vi "dfd_Modify NStage MRate Modeling.vi"(8 "error in (no error)":errorcluster, 11 "multirate filters in":T1[](array[typedef]) {"mMRate_SumWl" min=1 max=32 step=1; "mMRate_InputIwl" min=1 max=32 step=1; "mMRate_GainWl" min=1 max=32 step=1; "mMRate_OutputWl" min=1 max=32 step=1; "mMRate_InputWl" min=1 max=32 step=1; "mMRate_CoefWl" min=1 max=32 step=1; "mMRate_Mode" items=["Default"=-1, "No Rate Change"=0, "Interpolation"=1, "Decimation"=2, "Interpolated"=3, "Rational"=4]}) -> (0 "error out":errorcluster, 3 "multirate filters out":T1[](array[typedef]) {"mMRate_SumWl" min=1 max=32 step=1; "mMRate_InputIwl" min=1 max=32 step=1; "mMRate_GainWl" min=1 max=32 step=1; "mMRate_OutputWl" min=1 max=32 step=1; "mMRate_InputWl" min=1 max=32 step=1; "mMRate_CoefWl" min=1 max=32 step=1; "mMRate_Mode" items=["Default"=-1, "No Rate Change"=0, "Interpolation"=1, "Decimation"=2, "Interpolated"=3, "Rational"=4]})   [LabVIEW 2017, in "NI_DigFilter_FXP.lvlib"]
uses:
  <vilib>/addons/Digital Filter Design/NI_DigFilter_FXP.lvlib
  <vilib>/addons/Digital Filter Design/_Objects.llb/DFD Multirate Filter Obj.ctl
  <vilib>/addons/Digital Filter Design/_Objects.llb/DFD Multirate Mode.ctl
  <vilib>/addons/Digital Filter Design/_Objects.llb/DFD Coef Norm Type.ctl
  <vilib>/addons/Digital Filter Design/_Objects.llb/DFD Round-off Mode.ctl
  <vilib>/addons/Digital Filter Design/_Objects.llb/DFD FXP MRate Multiply Mode.ctl
  <vilib>/addons/Digital Filter Design/_Misc.llb/dfd_Error Handlers (Single).vi
  <vilib>/addons/Digital Filter Design/NI_DigFilterLicensed.lvlib
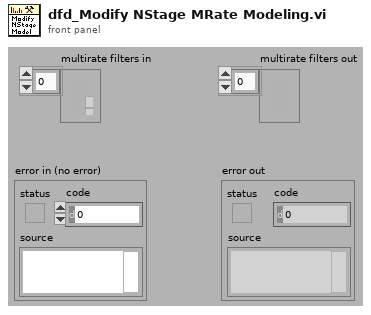
[diagram p1: front panel]
types:
  T1 = typedef "NI_DigFilterLicensed.lvlib/DFD Multirate Filter Obj.ctl" = cluster{"mMRate_Structure":enum16{"CIC", "FIR", "IIR", "Lattice"}, "mMRate_Mode":T2, "mMRate_Factor":i32, "mMRate_FIRParams":cluster{"mMRate_FIR_H":dbl[], "mMRate_FIR_IsNyquist?":bool, "mMRate_FIR_IsSymmetric?":bool}, "mMRate_CICParams":cluster{"mMRate_CIC_#Stage":i32, "mMRate_CIC_Lag":i32, "mMRate_CIC_Type":enum16{"Lowpass", "Highpass"}}, "mMRate_Order":i32, "mMRate_Version":string, "mMRate_Comments":string, "mMRate_RationalFactor":cluster{"mMRate_L":i32, "mMRate_M":i32}, "mMRate_Fs":dbl, "mMRate_Quantized?":bool, "mMRate_QFilterGain":dbl, "mMRate_CoefWl":i16, "mMRate_Scaling":cluster{"mMRate_ScaleByPowerOf2?":bool, "mMRate_ScaleType":T3}, "mMRate_InputWl":i16, "mMRate_OutputWl":i16, "mMRate_OutputMode":T4, "mMRate_MultMode":T5, "mMRate_BitPruning":bool, "mMRate_GainWl":i16, "mMRate_OutputFwl":i16, "mMRate_SumIwl":i16, "mMRate_InputIwl ":i16, "mMRate_SumWl":i16, "mMRate_CoefIwl":i16}
  T2 = typedef "NI_DigFilterLicensed.lvlib/DFD Multirate Mode.ctl" = i16
  T3 = typedef "NI_DigFilterLicensed.lvlib/DFD Coef Norm Type.ctl" = enum16{"No Norm", "Time Domain 1-Norm", "Time Domain 2-Norm", "Time Domain Inf-Norm"}
  T4 = typedef "NI_DigFilterLicensed.lvlib/DFD Round-off Mode.ctl" = enum16{"Nearest", "Truncation"}
  T5 = typedef "NI_DigFilterLicensed.lvlib/DFD FXP MRate Multiply Mode.ctl" = enum16{"Truncated", "Full"}
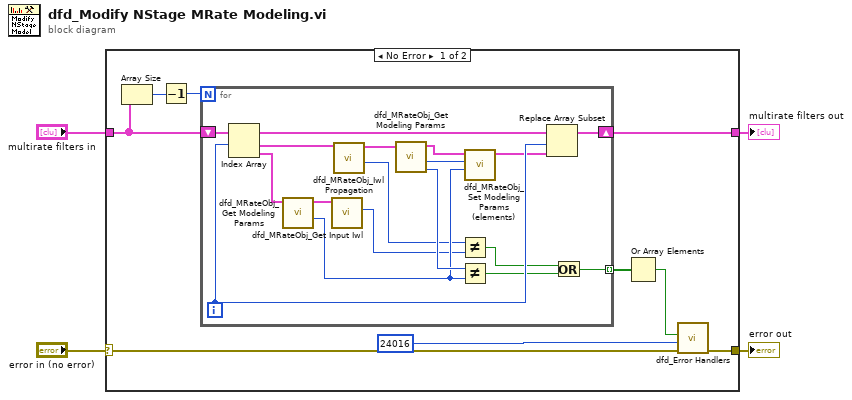
[diagram p0: block diagram]
diagram:
  n1 = case shown="No Error" "error in (no error)" {
    selector: "error in (no error)" -> [w5 w31]
    tunnel: [w13 _] -> w4
    tunnel: [w10 w31] -> w3
    tunnel: "multirate filters in" -> [w6 _]
    frame No Error {
      n2 = Array Size(array=w6) -> (size(s)=w12:i32)
      n3 = Decrement(x=w12) -> (x-1=w11:i32)
      n4 = for {
        N: w11 -> [_]
        shift-right: [w29] -> w13
        shift-left: w6 -> [w28]
        tunnel: [w18] -> w9 mode=indexing
        i -> [w27]
        n5 = Index Array(array=w28, index #1=w27) -> (element #1=w22:T1, element #2=w30:T1)  [unwired: 1 in]
        n6 = call <vilib>:"dfd_MRateObj_Get Modeling Params.vi"("multirate filter in"=w30) -> ("input wl"=w19:i16, "dup multirate filter"=w23:T1)  [unwired: 9 out]
        n7 = call <vilib>:"dfd_MRateObj_Get Input Iwl.vi"("multirate filter in"=w23) -> ("input iwl"=w14:i16)  [unwired: 10 out]
        n8 = call <vilib>:"dfd_MRateObj_Iwl Propagation.vi"("multirate filter"=w22) -> ("Actual Output iwl"=w16:i16, "dup multirate filter"=w21:T1)  [unwired: 9 out]
        n9 = call <vilib>:"dfd_MRateObj_Get Modeling Params.vi"("multirate filter in"=w21) -> ("output wl"=w25:i16, "input wl"=w26:i16, "dup multirate filter"=w20:T1)  [unwired: 8 out]
        n10 = Not Equal?(x=w16, y=w14) -> (x != y?=w17:bool)
        n11 = Not Equal?(x=w25, y=w19) -> (x != y?=w24:bool)
        n12 = call <vilib>:"dfd_MRateObj_Set Modeling Params (elements).vi"("output wl"=w19, "input wl"=w26, "multirate filter in"=w20) -> ("multirate filter out"=w15:T1)  [unwired: 1 in, 7 out]
        n13 = Replace Array Subset(array=w28, new element=w15, index=w27) -> (w29:T1[])
        n14 = Or(x=w17, y=w24) -> (x .or. y?=w18:bool)
      }
      n15 = Or Array Elements(Boolean array=w9) -> (logical OR=w8:bool)
      n16 = call-poly <vilib>:"dfd_Error Handlers.vi"("error in (no error)"=w5, "error code"=24016 ("WRN_IO_MODEL_INCONSISTENT"), "condition failed?"=w8) -> ("error out"=w10:errorcluster)  [unwired: 8 out]
    }
    frame Error {
    }
  }
  "error out" <- w3
  "multirate filters out" <- w4
